vi "SA_Init.vi"(8 "error in":errorcluster, 11 "VISA in":refnum<visa-resource-name>) -> (0 "error out":errorcluster, 3 "VISA out":refnum<visa-resource-name>)   [LabVIEW 2023, in "Keysight.lvlib"]
uses:
  Keysight.lvlib
panel:
  out "Keysight_FW_ver":string
  out "Keysight_SN":string
  out "Keysight_Model":string
  out "Keysight_Manufacturer":string
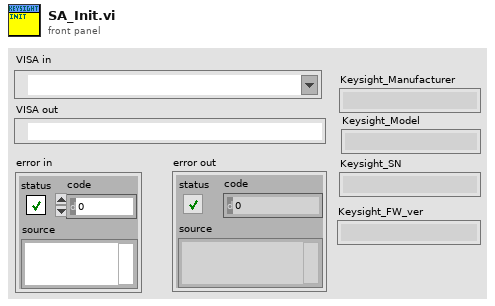
[diagram p1: front panel]
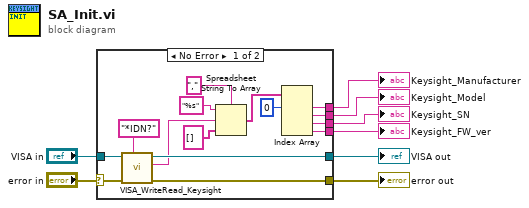
[diagram p0: block diagram]
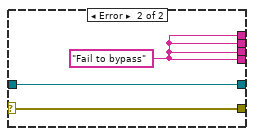
[diagram p2: hidden frame]
diagram:
  n1 = case shown="No Error" "error in" {
    selector: "error in" -> [w23 w25]
    tunnel: "VISA in" -> [w22 w26]
    tunnel: [w20 w25] -> w7
    tunnel: [w19 w26] -> w8
    tunnel: [w12 w24] -> w4
    tunnel: [w11 w24] -> w3
    tunnel: [w10 w24] -> w2
    tunnel: [w9 w24] -> w1
    frame No Error {
      n2 = call "VISA_WriteRead_Keysight.vi"("VISA_CMD"="*IDN?", "error in"=w23, "VISA in"=w22) -> ("error out"=w20:errorcluster, "Response"=w17:string, "VISA out"=w19:refnum<visa-resource-name>)  [unwired: 6 in]
      n3 = Spreadsheet String To Array(delimiter (Tab)=",", format string="%s", spreadsheet string=w17, array type (2D Dbl)=string[] []) -> (array=w14:string[])
      n4 = Index Array(array=w14, index #1=0 ("index")) -> (element #1=w12:string, element #2=w11:string, element #3=w10:string, element #4=w9:string)  [unwired: 3 in]
    }
    frame Error {
      w24 = "Fail to bypass" ("Response")
    }
  }
  "VISA out" <- w8
  "error out" <- w7
  "Keysight_Manufacturer" <- w4
  "Keysight_Model" <- w3
  "Keysight_SN" <- w2
  "Keysight_FW_ver" <- w1
